vi "Supported Smart Syntax Representation.vi"(0 "Message Popup in":refnum<class "DMM.lvclass">, 11 "error in (no error)":errorcluster) -> (4 "Message Popup out":refnum<class "DMM.lvclass">, 6 "Smart Syntax Representation List":string[](array[string]), 15 "error out":errorcluster)   [LabVIEW 2016, in "DMM.lvclass"]
uses:
  DMM.lvclass
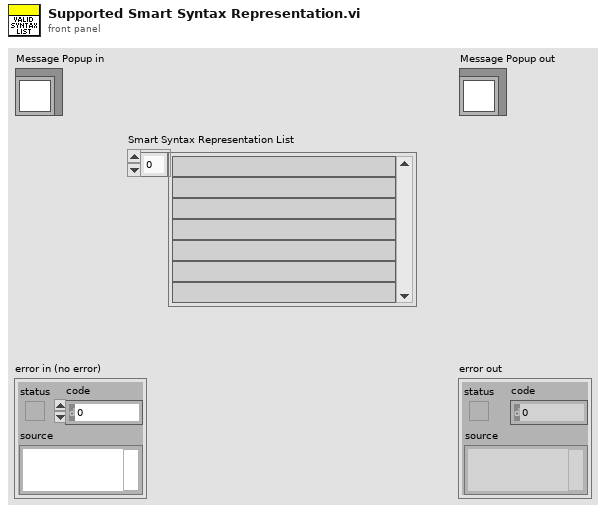
[diagram p1: front panel]
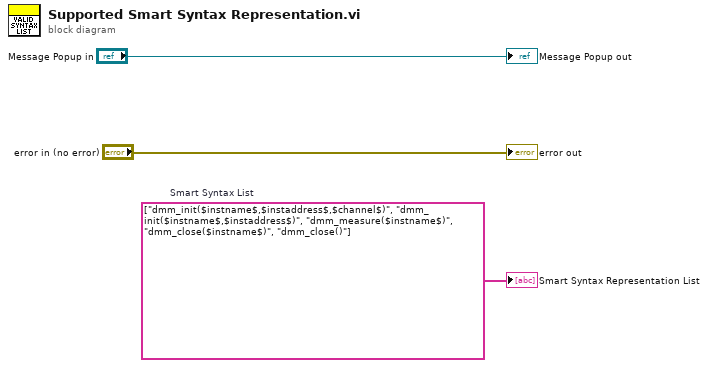
[diagram p0: block diagram]
diagram:
  w1 = string[] ["dmm_init($instname$,$instaddress$,$channel$)", "dmm_init($instname$,$instaddress$)", "dmm_measure($instname$)", "dmm_close($instname$)", "dmm_close()"]  # Smart Syntax List
  "error out" <- "error in (no error)"
  "Message Popup out" <- "Message Popup in"
  "Smart Syntax Representation List" <- w1
